vi "BuildCall.vi"(7 "PythonConverter_BD in":refnum<class "PyConvBD.lvclass">, 8 "error in":errorcluster, 11 "ForLoop in":refnum<class "ForLoop.lvclass">) -> (0 "error out":errorcluster, 3 "ForLoop out":refnum<class "ForLoop.lvclass">, 5 "PythonConverter_BD out":refnum<class "PyConvBD.lvclass">)   [LabVIEW 2014, in "Raspberry Pi Compatible Compiler for LabVIEW.lvlib" / "ForLoop.lvclass"]
uses:
  ForLoop.lvclass
  Python/PythonConverter_BD/PyConvBD.lvclass
  Python/Parsing/ListTypesTD.ctl
  Python/PythonConverter_BD/TypeDefs/NodeCall_TD.ctl
  Loop/Loop.lvclass/Loop.ctl
  ForLoop.lvclass/ForLoop.ctl
  ShiftRegister/ShiftRegister.lvclass/ShiftRegister.ctl
  Tunnel/Tunnel.lvclass
  RightShiftRegister/RightShiftRegister.lvclass
  LeftShiftRegister/LeftShiftRegister.lvclass
  LoopTunnel/LoopTunnel.lvclass
  Python/Parsing/Python Functions.lvlib
  Loop/Loop.lvclass
  ShiftRegister/ShiftRegister.lvclass
  Raspberry Pi Compatible Compiler for LabVIEW.lvlib
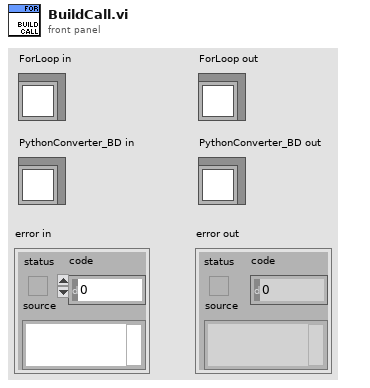
[diagram p1: front panel]
types:
  T1 = typedef "Raspberry Pi Compatible Compiler for LabVIEW.lvlib/NodeCall_TD.ctl" = cluster{"call":string, "collect":string, "Threaded":bool, "branches":string[]}
  T2 = typedef "Raspberry Pi Compatible Compiler for LabVIEW.lvlib/Python Functions.lvlib/ListTypesTD.ctl" = enum16{"list", "tuple", "parameter list", "output list", "return values"}
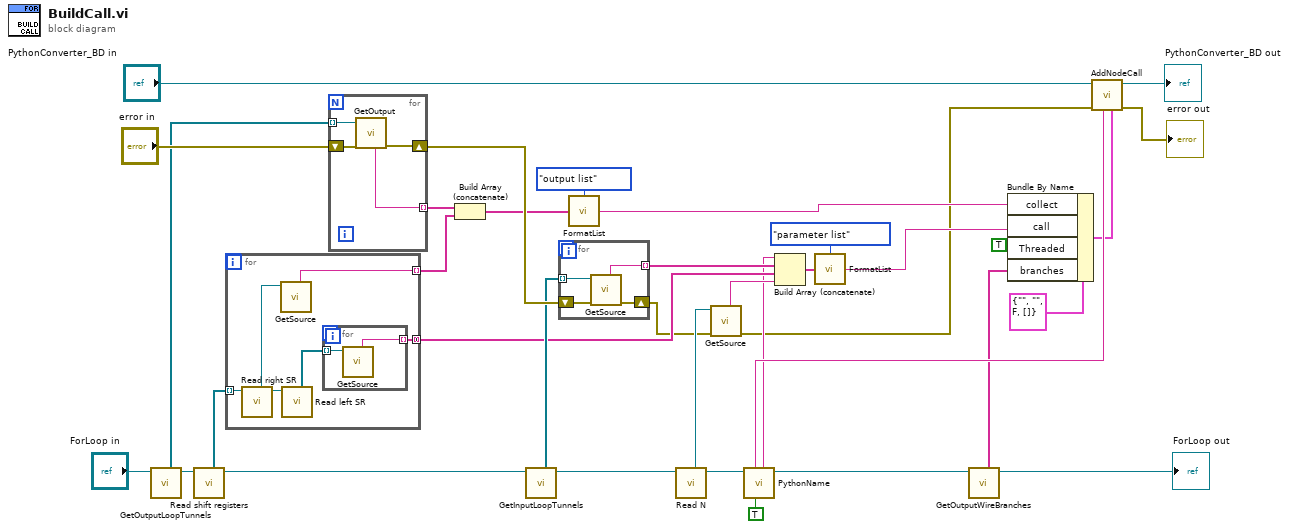
[diagram p0: block diagram]
diagram:
  n1 = call-dynamic "GetOutputLoopTunnels.vi"("Loop in"="ForLoop in") -> ("Loop out"=w18:refnum<class "ForLoop.lvclass">, "tunnels"=w21:refnum<class "LoopTunnel.lvclass">[])  [unwired: 6 in, 1 out]
  n2 = call "Read shift registers.vi"("Loop in"=w18) -> ("Loop out"=w17:refnum<class "ForLoop.lvclass">, "shift registers"=w16:refnum<class "ShiftRegister.lvclass">[])  [unwired: 7 in]
  n3 = for {
    tunnel: w16 -> [w42] mode=indexing
    tunnel: [w40] -> w14 mode=indexing
    tunnel: [w37] -> w12 mode=concatenating
    n4 = call "Read right SR.vi"("ShiftRegister in"=w42) -> ("ShiftRegister out"=w39:refnum<class "ShiftRegister.lvclass">, "right SR"=w41:refnum<class "RightShiftRegister.lvclass">)  [unwired: 7 in]
    n5 = call-dynamic "GetSource.vi"("RightShiftRegister in"=w41) -> ("name"=w40:string)  [unwired: 6 in, 2 out]
    n6 = call "Read left SR.vi"("ShiftRegister in"=w39) -> ("left SR"=w38:refnum<class "LeftShiftRegister.lvclass">[])  [unwired: 7 in, 1 out]
    n7 = for {
      tunnel: w38 -> [w44] mode=indexing
      tunnel: [w43] -> w37 mode=indexing
      n8 = call-dynamic "GetSource.vi"("LeftShiftRegister in"=w44) -> ("name"=w43:string)  [unwired: 6 in, 2 out]
    }
  }
  n9 = for {
    tunnel: w21 -> [w48] mode=indexing
    shift-right: [w45] -> w32
    shift-left: "error in" -> [w47]
    tunnel: [w46] -> w36 mode=indexing
    n10 = call-dynamic "GetOutput.vi"("error in"=w47, "Tunnel in"=w48) -> ("error out"=w45:errorcluster, "name"=w46:string)  [unwired: 5 in, 1 out]
  }
  n11 = Build Array (concatenate)(w36, w14) -> (w15:string[])
  n12 = call-dynamic "GetInputLoopTunnels.vi"("Loop in"=w17) -> ("Loop out"=w19:refnum<class "ForLoop.lvclass">, "tunnels"=w20:refnum<class "LoopTunnel.lvclass">[])  [unwired: 6 in, 1 out]
  n13 = for {
    tunnel: w20 -> [w52] mode=indexing
    shift-right: [w50] -> w5
    shift-left: w32 -> [w51]
    tunnel: [w49] -> w25 mode=indexing
    n14 = call-dynamic "GetSource.vi"("error in"=w51, "Tunnel in"=w52) -> ("error out"=w50:errorcluster, "name"=w49:string)  [unwired: 5 in, 1 out]
  }
  n15 = call "FormatList.vi"("values"=w15, "type"=ListTypesTD."output list") -> ("python object"=w6:string)
  n16 = call "Read N.vi"("ForLoop in"=w19) -> ("ForLoop out"=w26:refnum<class "ForLoop.lvclass">, "N"=w23:refnum<class "Tunnel.lvclass">)  [unwired: 7 in]
  n17 = call-dynamic "GetSource.vi"("error in"=w5, "Tunnel in"=w23) -> ("error out"=w4:errorcluster, "name"=w13:string)  [unwired: 5 in, 1 out]
  n18 = call-dynamic "PythonName.vi"("add self"=TRUE, "Node in"=w26) -> ("Node out"=w3:refnum<class "ForLoop.lvclass">, "name"=w7:string, "UID"=w33:string)  [unwired: 6 in, 1 out]
  n19 = Build Array (concatenate)(w7, w25, w12, w13) -> (w24:string[])
  n20 = call "FormatList.vi"("values"=w24, "type"=ListTypesTD."parameter list") -> ("python object"=w9:string)
  n21 = call-dynamic "GetOutputWireBranches.vi"("Loop in"=w3) -> ("Loop out"=→"ForLoop out":refnum<class "ForLoop.lvclass">, "branches"=w1:string[])  [unwired: 6 in, 1 out]
  n22 = Bundle By Name(cluster=T1 {"call"="", "collect"="", "Threaded"=FALSE, "branches"=[]} ("call"), "collect"=w6, "call"=w9, "Threaded"=TRUE, "branches"=w1) -> (w8:T1)
  n23 = call "AddNodeCall.vi"("call"=w8, "name"=w33, "error in"=w4, "PythonConverter_BD in"="PythonConverter_BD in") -> ("error out"=→"error out":errorcluster, "PythonConverter_BD out"=→"PythonConverter_BD out":refnum<class "PyConvBD.lvclass">)  [unwired: 4 in]
